vi "UDP Size Mismatch Error.vi"(7 "source vi name":string, 8 "error in (no error)":errorcluster, 9 "actual size":u64, 10 "expected size":u64, 11 "UDP in":refnum<class "UDP Transceiver.lvclass">) -> (0 "error out":errorcluster, 3 "UDP out":refnum<class "UDP Transceiver.lvclass">)   [LabVIEW 2017, in "UDP.lvlib" / "UDP Transceiver.lvclass"]
uses:
  UDP Transceiver.lvclass
  Errors.ctl
  <vilib>/NI/Memory Manager/VIs/Write Numeric Scalar to Source (Base10 U64).vi
  <vilib>/NI/Memory Manager/Static Errors.lvlib
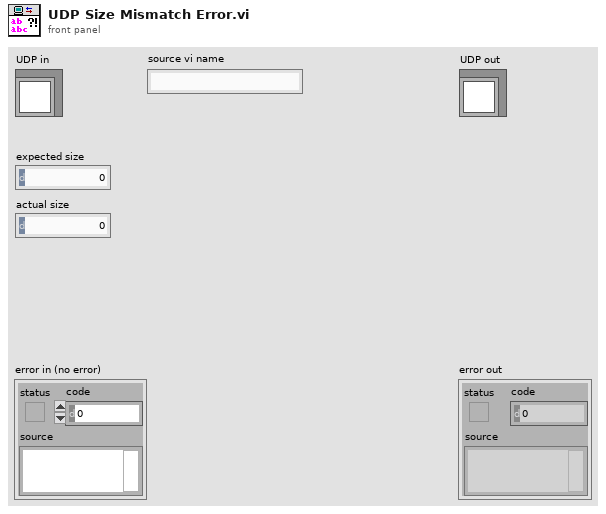
[diagram p1: front panel]
types:
  T1 = typedef "UDP.lvlib/UDP Transceiver.lvclass/Errors.ctl" = enum16{"Unknown Datagram", "Size Mismatch"}
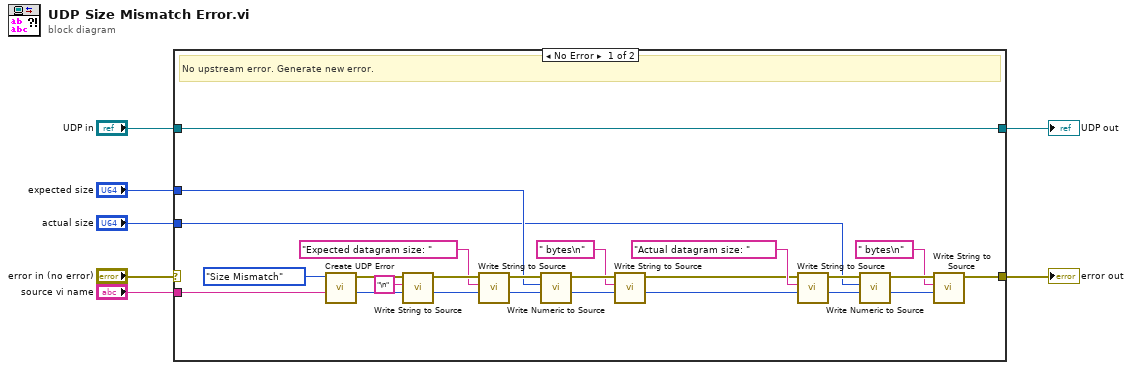
[diagram p0: block diagram]
diagram:
  n1 = case shown="No Error" "error in (no error)" {
    selector: "error in (no error)" -> [_ w33]
    tunnel: [w11 w33] -> w2
    tunnel: "UDP in" -> [w10 w34]
    tunnel: [w10 w34] -> w1
    tunnel: "actual size" -> [w9 _]
    tunnel: "expected size" -> [w22 _]
    tunnel: "source vi name" -> [w32 _]
    frame No Error {
      # "No upstream error. Generate new error."
      n2 = call "Create UDP Error.vi"("source vi name"=w32, "Error"=Errors."Size Mismatch") -> ("offset"=w30:i32, "error out"=w28:errorcluster)  [unwired: 8 in]
      n3 = call <vilib>:"Write String to Source.vi"("offset"=w30, "string"="\n", "error in"=w28) -> ("new offset"=w26:i32, "error out"=w27:errorcluster)  [unwired: 7 in]
      n4 = call <vilib>:"Write String to Source.vi"("offset"=w26, "string"="Expected datagram size: ", "error in"=w27) -> ("new offset"=w23:i32, "error out"=w24:errorcluster)  [unwired: 7 in]
      n5 = call-poly <vilib>:"Write Numeric to Source.vi"("offset"=w23, "value"=w22, "error in"=w24) -> ("new offset"=w20:i32, "error out"=w21:errorcluster)  [unwired: 7 in]
      n6 = call <vilib>:"Write String to Source.vi"("offset"=w20, "string"=" bytes\n", "error in"=w21) -> ("new offset"=w12:i32, "error out"=w13:errorcluster)  [unwired: 7 in]
      n7 = call <vilib>:"Write String to Source.vi"("offset"=w12, "string"="Actual datagram size: ", "error in"=w13) -> ("new offset"=w16:i32, "error out"=w15:errorcluster)  [unwired: 7 in]
      n8 = call-poly <vilib>:"Write Numeric to Source.vi"("offset"=w16, "value"=w9, "error in"=w15) -> ("new offset"=w18:i32, "error out"=w17:errorcluster)  [unwired: 7 in]
      n9 = call <vilib>:"Write String to Source.vi"("offset"=w18, "string"=" bytes\n", "error in"=w17) -> ("error out"=w11:errorcluster)  [unwired: 7 in, 1 out]
    }
    frame Error {
      # "Upstream error. Pass through."
    }
  }
  "error out" <- w2
  "UDP out" <- w1
